vi "Table, Set Column Value, Double.vi"(6 "column (0)":i32, 7 "format (%f)":string="%f", 8 "error in":errorcluster, 10 "Value":dbl[](array[numeric]), 11 "Tbl Refnum":refnum<vi>) -> (0 "error out":errorcluster, 3 "Tbl Refnum out":refnum<vi>, 4 "column+1":i32)   [LabVIEW 2010]
doc: "This function writes an Array of Doubles to a table column."
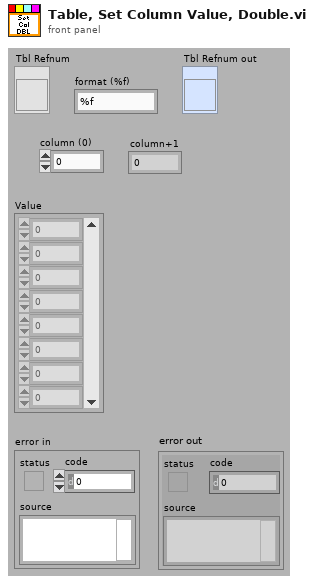
[diagram p1: front panel]
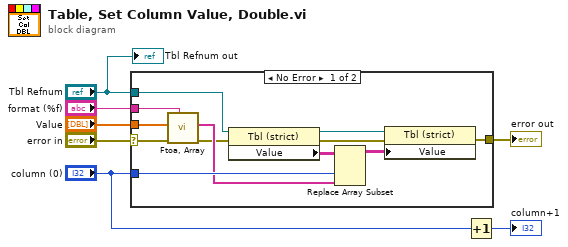
[diagram p0: block diagram]
diagram:
  n1 = case shown="No Error" "error in" {
    selector: "error in" -> [w9 w20]
    tunnel: "Tbl Refnum" -> [w19 _]
    tunnel: [w18 w20] -> w7
    tunnel: "column (0)" -> [w14 _]
    tunnel: "Value" -> [w12 _]
    tunnel: "format (%f)" -> [w8 _]
    frame No Error {
      n2 = call "Ftoa, Array.vi"("format (%f)"=w8, "error in"=w9, "value"=w12) -> ("error out"=w10:errorcluster, "string"=w11:string[])  [unwired: 5 in]
      n3 = property class="Tbl (strict)"(reference=w19, error in=w10) -> (reference out=w13:refnum<vi>, error out=w17:errorcluster, "Value"=w15:string[][])
      n4 = Replace Array Subset(array=w15, new element=w11, index (col)=w14) -> (w16:string[][])  [unwired: 1 in]
      n5 = property class="Tbl (strict)"(reference=w13, error in=w17, "Value"=w16) -> (error out=w18:errorcluster)  [unwired: 1 out]
    }
    frame Error {
    }
  }
  "error out" <- w7
  n6 = Increment(x="column (0)") -> (x+1=→"column+1":i32)
  "Tbl Refnum out" <- "Tbl Refnum"
